vi "Create.vi"(8 "error in (no error)":errorcluster) -> (0 "error out":errorcluster, 3 "Simulated Serial":refnum<class "Simulated Serial.lvclass">)   [LabVIEW 2020, in "Simulated Serial.lvclass"]
uses:
  Simulated Serial.lvclass
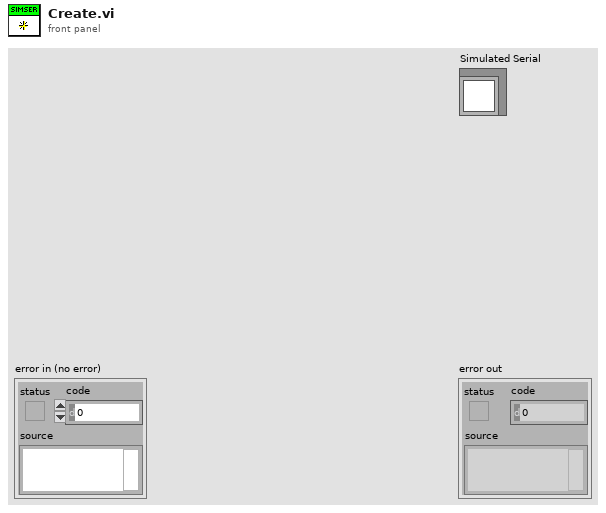
[diagram p1: front panel]
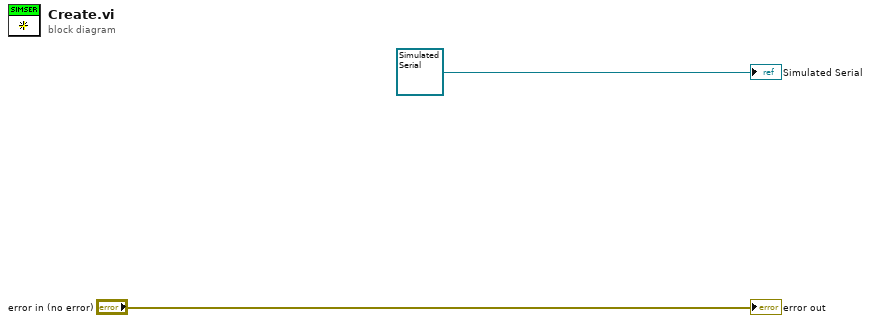
[diagram p0: block diagram]
diagram:
  "error out" <- "error in (no error)"
  "Simulated Serial" <- refnum<class "Simulated Serial.lvclass"> refnum ("Simulated Serial")
